vi "DO TEST.vi"() -> ()   [LabVIEW 2018]
uses:
  <vilib>/DAQmx/read.llb/DAQmx Read (Digital 1D Bool NChan 1Samp 1Line).vi
  <vilib>/DAQmx/write.llb/DAQmx Write (Digital 1D Bool NChan 1Samp 1Line).vi
panel:
  in  "按钮":bool
  in  "data 2":bool[](array[boolean]) caption="数据"
  out "data":bool[](array[boolean]) caption="数据"
  in  "Digital Output Array":T1(array[cluster])
  in  "索引":i32
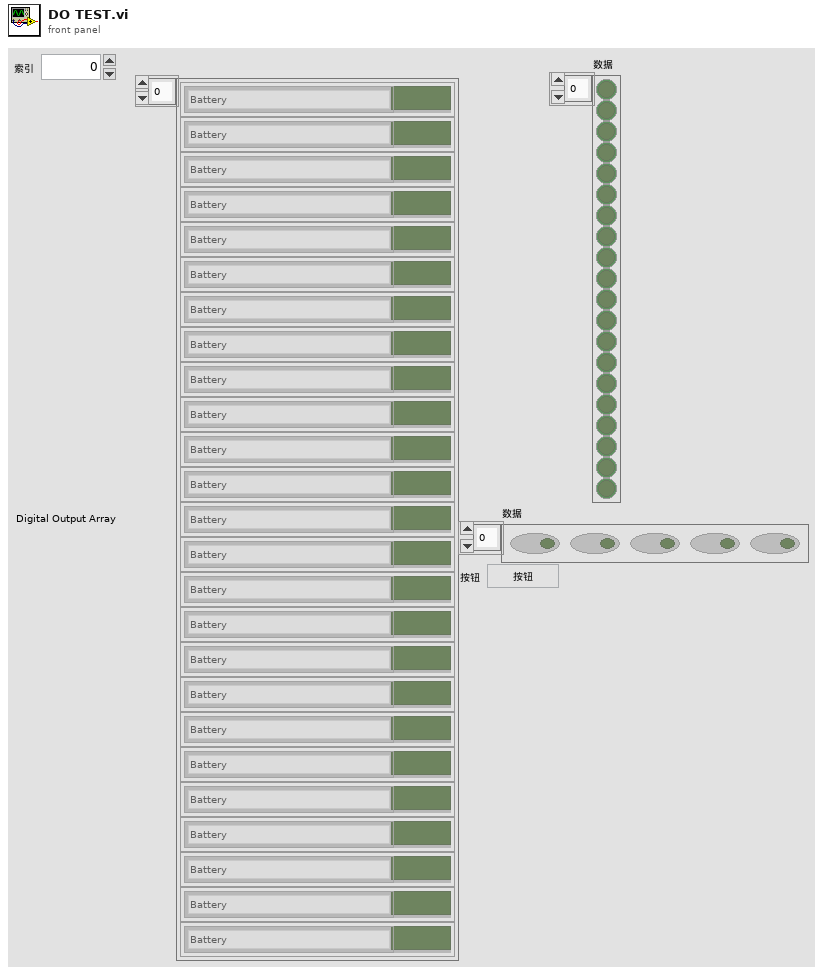
[diagram p1: front panel]
types:
  T1 = cluster{"Status":bool, "Global DO Ch":enum16{"Battery", "Ignition High", "Switch 1", "Switch 2", "Switch 3", "Select NI LIN", "Prerun Switch 4", "Prerun Switch 5", "Prerun Switch 6", "Prerun Ignition Low", "Prerun Glass Analog Switch 1", "Prerun Glass Analog Switch 2", "Prerun Glass Analog Switch 3", "Prerun Glass Analog Switch 4", "Prerun Sunshade Analog Switch 1", "Prerun Sunshade Analog Switch 2", "Prerun Sunshade Analog Switch 3", "Prerun Sunshade Analog Switch 4", "Prerun Select RS232 LIN", "Prerun Select RS232", "Prerun Select CAN", "Prerun Park/Enable", "Prerun Communications Power", "Prerun BMW Glass Motor Relay 1", "Prerun BMW Glass Motor Relay 2", "Prerun BMW Sunshade Motor Relay 1", "Prerun BMW Sunshade Motor Relay 2", "Prerun Spare 1", "Prerun Spare 2", "Prerun Spare 3", "Prerun Spare 4", "Prerun Spare 5", "Audit Battery", "Audit Ignition High", "Audit Ignition Low", "Audit Switch 1", "Audit Switch 2", "Audit Switch 3", "Audit Switch 4", "Audit Switch 5", "Audit Switch 6", "Audit Glass Analog Switch 1", "Audit Glass Analog Switch 2", "Audit Glass Analog Switch 3", "Audit Glass Analog Switch 4", "Audit Sunshade Analog Switch 1", "Audit Sunshade Analog Switch 2", "Audit Sunshade Analog Switch 3", "Audit Sunshade Analog Switch 4", "Audit Select NI LIN", "Audit Select RS232 LIN", "Audit Select RS232", "Audit Select CAN", "Audit Park/Enable", "Audit Communications Power", "Audit BMW Glass Motor Relay 1", "Audit BMW Glass Motor Relay 2", "Audit BMW Sunshade Motor Relay 1", "Audit BMW Sunshade Motor Relay 2", "Audit Spare 1", "Audit Spare 2", "Audit Spare 3", "Audit Spare 4", "Audit Spare 5", "Repair Battery", "Repair Ignition High", "Repair Switch 1", "Repair Switch 2", "Repair Select NI LIN", "Repair Ignition Low", "Repair Switch 3", "Repair Switch 4", "Repair Switch 5", "Repair Switch 6", "Repair Glass Analog Switch 1", "Repair Glass Analog Switch 2", "Repair Glass Analog Switch 3", "Repair Glass Analog Switch 4", "Repair Sunshade Analog Switch 1", "Repair Sunshade Analog Switch 2", "Repair Sunshade Analog Switch 3", "Repair Sunshade Analog Switch 4", "Repair Select RS232 LIN", "Repair Select RS232", "Repair Select CAN", "Repair Select Park/Enable", "Repair Communications Power", "Repair BMW Glass Motor Relay 1", "Repair BMW Glass Motor Relay 2", "Repair BMW Sunshade Motor Relay 1", "Repair BMW Sunshade Motor Relay 2", "Repair Spare 1", "Repair Spare 2", "Repair Spare 3", "Repair Spare 4", "Repair Spare 5", "Breakin Battery", "Breakin Igntiion High", "Breakin Ignition Low", "Breakin Switch 1", "Breakin Switch 2", "Breakin Switch 3", "Breakin Switch 4", "Breakin Switch 5", "Breakin Switch 6", "Breakin Glass Analog Switch 1", "Breakin Glass Analog Switch 2", "Breakin Glass Analog Switch 3", "Breakin Glass Analog Switch 4", "Breakin Sunshade Analog Switch 1", "Breakin Sunshade Analog Switch 2", "Breakin Sunshade Analog Switch 3", "Breakin Sunshade Analog Switch 4", "Breakin Select NI LIN", "Breakin Select RS232 LIN", "Breakin Select RS232", "Breakin Select CAN", "Breakin Park/Enable", "Breakin Communications Power", "Breakin BMW Glass Motor Relay 1", "Breakin BMW Glass Motor Relay 2", "Breakin BMW Sunshade Motor Relay 1", "Breakin BMW Sunshade Motor Relay 2", "Breakin Spare 1", "Breakin Spare 2", "Breakin Spare 3", "Breakin Spare 4", "Breakin Spare 5", "Not Implemented"}}[]
  T2 = enum16{"Init", "Write", "Write All", "Clear All", "Stop", "Read"}
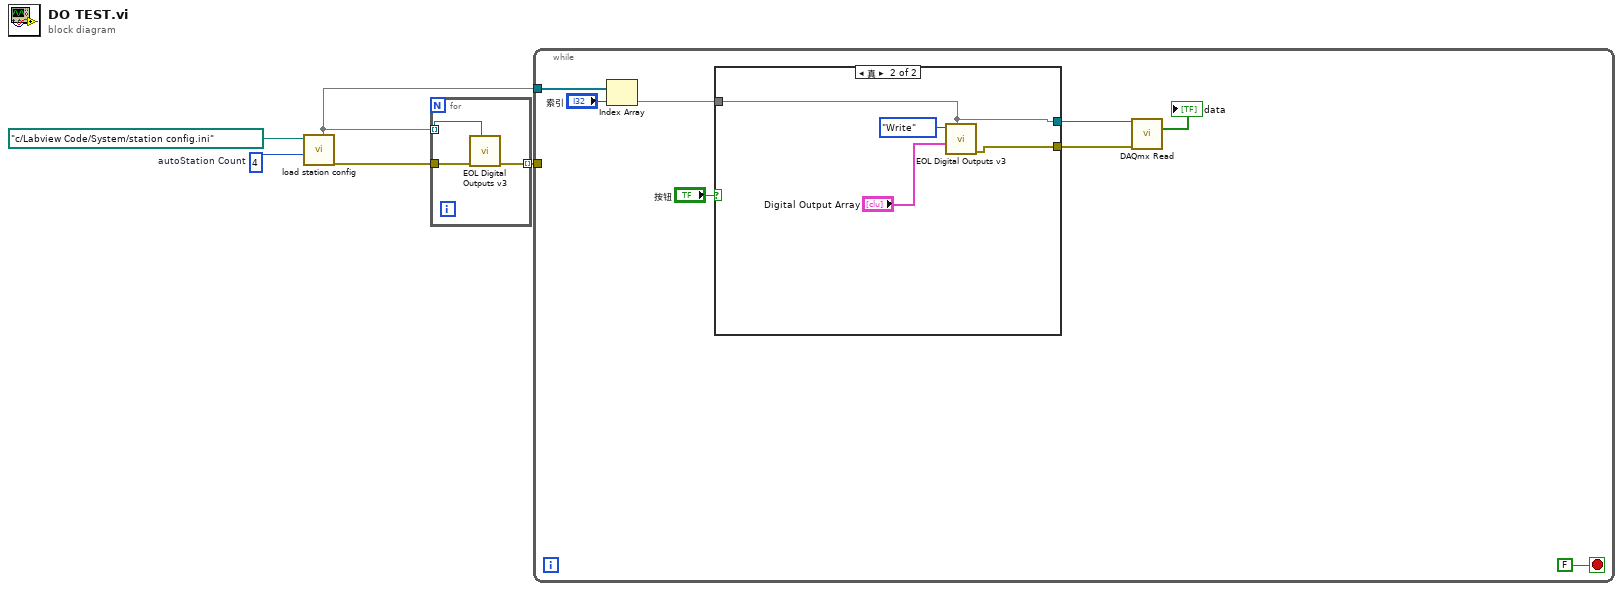
[diagram p0: block diagram]
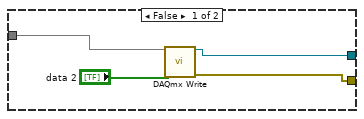
[diagram p2: hidden frame]
diagram:
  w4 = 4  # autoStation Count
  n1 = call "load station config.vi"(10:w4, "station config file path"=path "c:/Labview Code/System/station config.ini") -> ("error out"=w3:errorcluster, 5:w1)  [unwired: 6 in, 2 out]
  n2 = for {
    tunnel: w3 -> [w8]
    tunnel: w1 -> [w7] mode=indexing
    tunnel: [w6] -> w2 mode=indexing
    n3 = call "EOL Digital Outputs v3.vi"("task/channels in"=w7, "Error In"=w8) -> ("Error Out"=w6:errorcluster)  [unwired: 8 in, 1 out]
  }
  n4 = while {
    tunnel: w2 -> [_]
    tunnel: w1 -> [w16]
    stop <- FALSE stop-if-true
    n5 = Index Array(array=w16, index="索引") -> (element=w14)
    n6 = case shown="真" "按钮" {
      tunnel: w14 -> [w20 w21]
      tunnel: [w17 w24] -> w13
      tunnel: [w18 w21] -> w10
      frame False {
        n7 = call-poly <vilib>:"DAQmx Write.vi"("task/channels in"=w20, "data"="data 2") -> ("task out"=w18:refnum<k21>, "error out"=w17:errorcluster)  [unwired: 11 in, 1 out]
      }
      frame True {
        n8 = call "EOL Digital Outputs v3.vi"("task/channels in"=w21, "DO Status"="Digital Output Array", "Mode"=T2."Write") -> ("Error Out"=w24:errorcluster)  [unwired: 7 in, 1 out]
      }
    }
    n9 = call-poly <vilib>:"DAQmx Read.vi"("task/channels in"=w10, "error in"=w13) -> ("data"=→"data":bool[])  [unwired: 11 in, 2 out]
  }
